vi "asyncMaxSearch.vi"(6 "reset":bool, 7 "enable":bool, 9 "maxSearchBounds":T1={"maxSearchUpper"=600, "maxSearchLower"=200}, 11 "inputPair":cluster{"index":u16, "data":i16}) -> (0 "outputValid":bool, 3 "output":cluster{"index":u16, "data":i16})   [LabVIEW 2016]
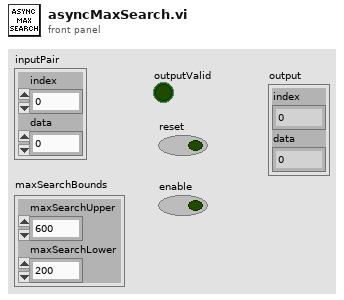
[diagram p1: front panel]
types:
  T1 = cluster{"maxSearchUpper":u16, "maxSearchLower":u16}
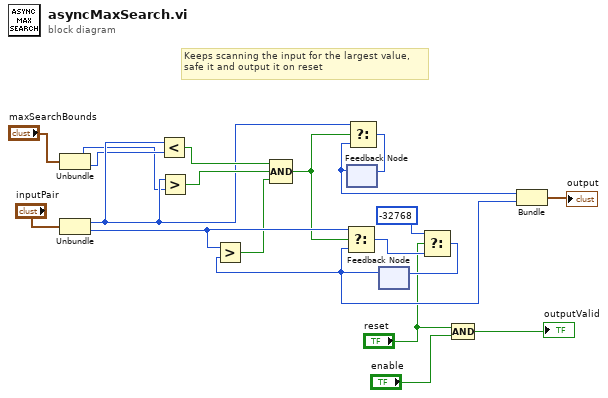
[diagram p0: block diagram]
diagram:
  # "Keeps scanning the input for the largest value,\nsafe it and output it on reset"
  n1 = Unbundle("maxSearchBounds") -> ("maxSearchUpper"=w1:u16, "maxSearchLower"=w2:u16)
  n2 = Unbundle("inputPair") -> ("index"=w14:u16, "data"=w16:i16)
  n3 = Less?(x=w14, y=w2) -> (x < y?=w18:bool)
  n4 = Greater?(x=w14, y=w1) -> (0:w17:bool)
  n5 = feedback #1() -> (w10:u16)  [unwired: 1 in]
  n6 = feedback #2() -> (w9:i16)  [unwired: 1 in]
  n7 = Greater?(x=w16, y=w9) -> (0:w6:bool)
  n8 = Compound Arithmetic op=AND(w18, w17, w6) -> (w5:bool)
  n9 = Select(t=w16, s=w5, f=w9) -> (s? t:f=w13:i16)
  n10 = Select(t=w14, s=w5, f=w10) -> (s? t:f=w15:u16)
  n11 = feedback-in #1(w15) -> ()
  n12 = Select(t=i16 -32768, s="reset", f=w13) -> (s? t:f=w11:i16)
  n13 = feedback-in #2(w11) -> ()
  n14 = Compound Arithmetic op=AND("reset", "enable") -> (→"outputValid":bool)
  n15 = Bundle("index"=w10, "data"=w9) -> (→"output":cluster{"index":u16, "data":i16})  [unwired: 1 in]
